vi "PicoLogHRDLGetSingleAsyncExample.vi"() -> ()   [LabVIEW 2010]
panel:
  out "maxAdc":i32
  out "Over Voltage":i16 format="%016b"
  out "handle":i16
  out "error out":errorcluster
  out "Unit Info":T1
  in  "range":i16=-1
  in  "channel":i16=-1
  in  "value":i32
  out "bStartedConversion":bool
  out "bConversionFinished":bool
  in  "stop":bool
  in  "error in (no error)":errorcluster
  out "Meter (mV)":dbl(knob)=-inf scale=-2500.0..2500.0
  in  "Input type":i16(ring)=1 items=["Differential", "Single-Ended"]
  in  "Conversion time":i16(ring)=4 items=["60ms", "100ms", "180ms", "340ms", "660ms"]
  in  "Voltage Range":i16(ring) items=["+/-2500mV", "+/-1200mV", "+/-625mV", "+/-312.5mV", "+/-156.25mV", "+/-78.125mV", "+/-39.0625mV"]
  in  "Channel":i16=1 min=1 max=16 step=1
  # "-1        if the unit fails to open\n0         if no unit is found\n>= 1   handle to the device opened"
  # "NOTES-\nNumber of channels-\nADC-20: 1 to 8\nADC-24: 1 to 16\n\nRange Voltage range Availability\n (0)    ±2500 mV        ADC-20 and ADC-24\n (1)    ±1250 mV        ADC-20 and ADC-24\n (2)    ±625 mV          ADC-24 only\n (3)    ±312.5 mV       ADC-24 only\n (4)    ±156.25 mV     ADC-24 only\n (5)    ±78.125 mV     ADC-24 only\n (6)    ±39.0625 mV   ADC-24 only"
  # "mV"
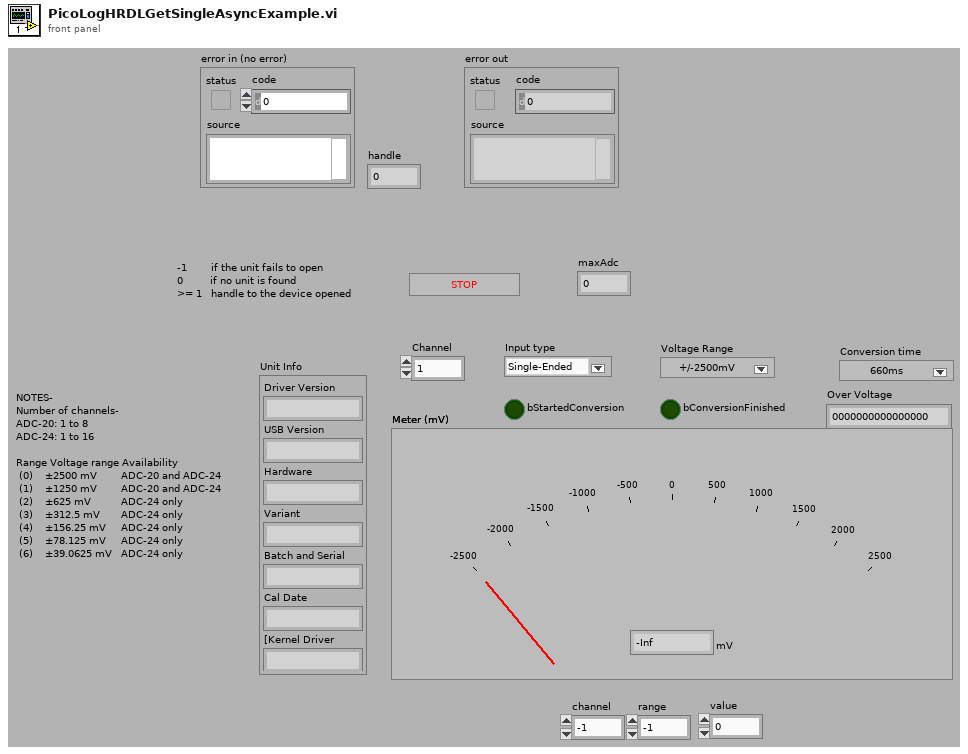
[diagram p1: front panel]
types:
  T1 = cluster{"Driver Version":string, "USB Version":string, "Hardware":string, "Variant":string, "Batch and Serial":string, "Cal Date":string, "[Kernel Driver":string, "[7]":string, "[8]":string, "[9]":string, "[10]":string, "[11]":string, "[12]":string, "[13]":string, "[14]":string}
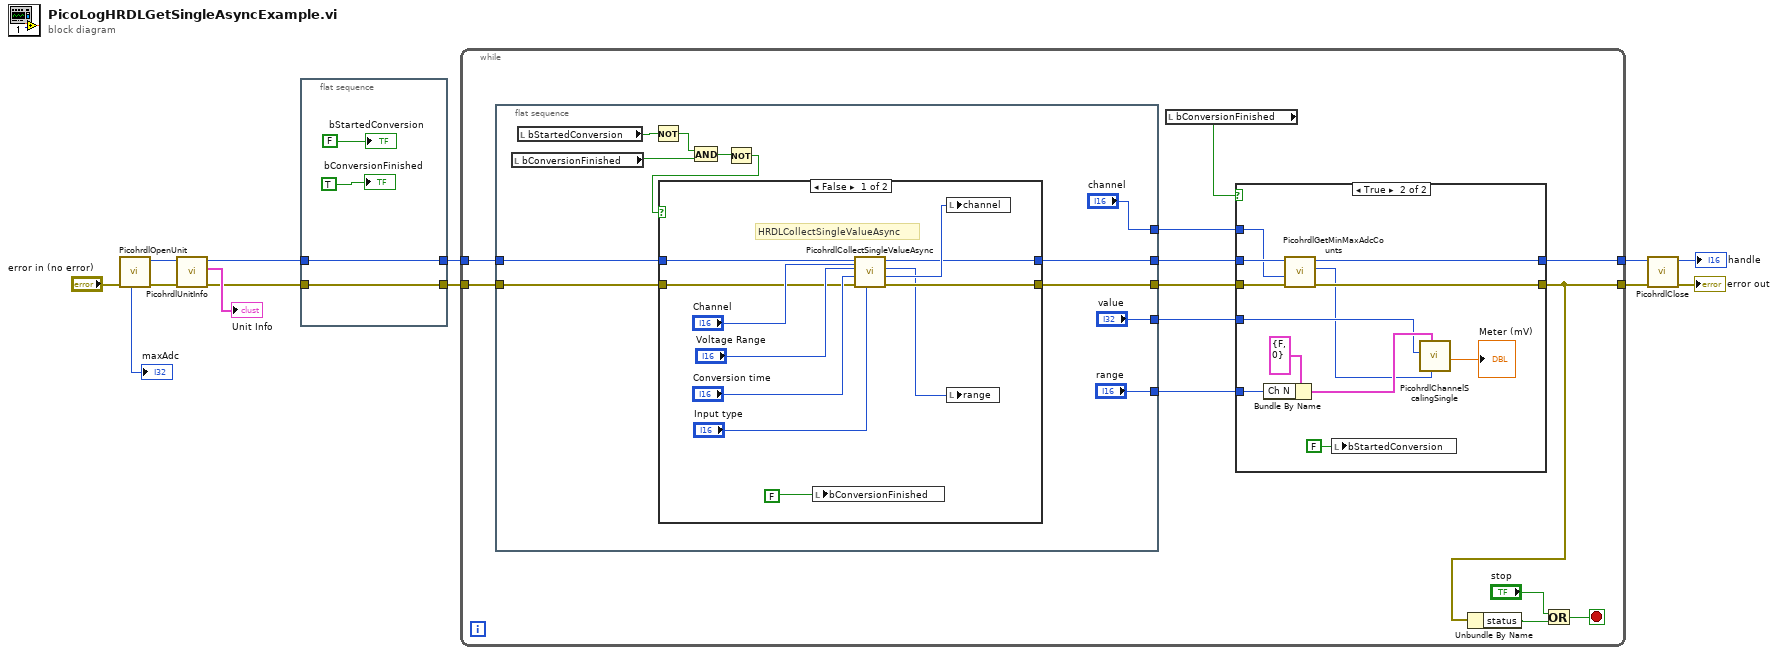
[diagram p0: block diagram]
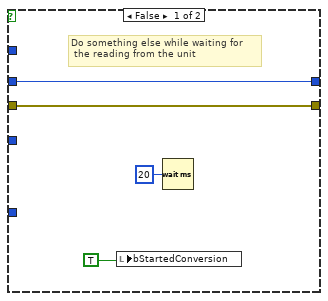
[diagram p2: hidden frame]
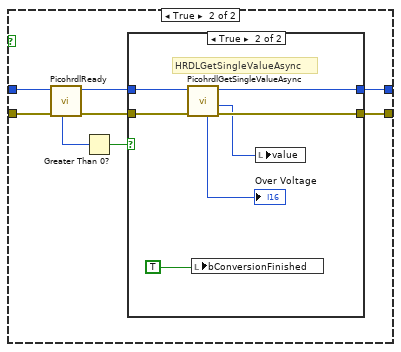
[diagram p3: hidden frame]
diagram:
  n1 = call "PicohrdlOpenUnit.vi"("error in (no error)"="error in (no error)") -> ("error out"=w11:errorcluster, "Handle out"=w10:i16, "maxAdc"=→"maxAdc":i32)  [unwired: 7 in, 1 out]
  n2 = call "PicohrdlUnitInfo.vi"("error in (no error)"=w11, "handle in"=w10) -> ("error out"=w4:errorcluster, "Unit Info"=→"Unit Info":T1, "handle out"=w2:i16)  [unwired: 7 in]
  n3 = flat-sequence {
    tunnel: [w15] -> w5
    tunnel: w4 -> [w15]
    tunnel: [w14] -> w3
    tunnel: w2 -> [w14]
    frame #0 {
      "bStartedConversion" <- FALSE ("bStartedConversion")
      "bConversionFinished" <- TRUE ("bConversionFinished")
    }
  }
  n4 = while {
    tunnel: w3 -> [w25]
    tunnel: [w23] -> w6
    tunnel: [w19] -> w7
    tunnel: w5 -> [w20]
    stop <- w28 stop-if-true
    n5 = flat-sequence {
      tunnel: ["range"] -> w27
      tunnel: ["value"] -> w26
      tunnel: w25 -> [w58]
      tunnel: [w57] -> w24
      tunnel: ["channel"] -> w22
      tunnel: [w56] -> w21
      tunnel: w20 -> [w55]
      frame #0 {
        n6 = local read "bConversionFinished"() -> (w51:bool)
        n7 = local read "bStartedConversion"() -> (w48:bool)
        n8 = Not(x=w48) -> (.not. x?=w47:bool)
        n9 = And(x=w47, y=w51) -> (x .and. y?=w50:bool)
        n10 = Not(x=w50) -> (.not. x?=w49:bool)
        n11 = case shown="False" w49 {
          tunnel: w58 -> [w60 w70]
          tunnel: [w61 w76] -> w57
          tunnel: [w64 w75] -> w56
          tunnel: w55 -> [w59 w74]
          frame False {
            # "HRDLCollectSingleValueAsync"
            n12 = local write "bConversionFinished"(FALSE ("bStartedConversion")) -> ()
            n13 = call "PicohrdlCollectSingleValueAsync.vi"("Input type"="Input type", "Channel in"="Channel", "error in (no error)"=w59, "Conversion time"="Conversion time", "Voltage Range"="Voltage Range", "handle in"=w60) -> ("error out"=w64:errorcluster, "channel"=w63:i16, "Voltage Range out"=w62:i16, "Handle out"=w61:i16)  [unwired: 2 in]
            n14 = local write "channel"(w63) -> ()
            n15 = local write "range"(w62) -> ()
          }
          frame True {
            n16 = call "PicohrdlReady.vi"("error in (no error)"=w74, "handle in"=w70) -> ("error out"=w73:errorcluster, "handle out"=w71:i16, "ready"=w72:i16)  [unwired: 7 in]
            n17 = Greater Than 0?(x=w72) -> (x > 0?=w77:bool)
            n18 = case shown="True" w77 {
              tunnel: w71 -> [w79 w84]
              tunnel: w73 -> [w78 w85]
              tunnel: [w79 w82] -> w76
              tunnel: [w78 w83] -> w75
              frame False {
                # "Unit still not ready"
              }
              frame True {
                # "HRDLGetSingleValueAsync"
                n19 = call "PicohrdlGetSingleValueAsync.vi"("error in (no error)"=w85, "handle in"=w84) -> ("error out"=w83:errorcluster, "value"=w80:i32, "Handle out"=w82:i16, "Over Voltage"=→"Over Voltage":i16)  [unwired: 6 in]
                n20 = local write "bConversionFinished"(TRUE ("bConversionFinished")) -> ()
                n21 = local write "value"(w80) -> ()
              }
            }
          }
        }
      }
    }
    n22 = local read "bConversionFinished"() -> (w30:bool)
    n23 = case shown="True" w30 {
      tunnel: w27 -> [_ w44]
      tunnel: w26 -> [_ w42]
      tunnel: w24 -> [w34 w40]
      tunnel: [w34 w36] -> w23
      tunnel: w22 -> [_ w38]
      tunnel: [w33 w37] -> w19
      tunnel: w21 -> [w33 w39]
      frame False {
        # "Do something else while waiting for\n the reading from the unit"
        n24 = local write "bStartedConversion"(TRUE ("bStartedConversion")) -> ()
        n25 = Wait (ms)(milliseconds to wait=u32 20) -> ()  [unwired: 1 out]
      }
      frame True {
        n26 = Bundle By Name(cluster=cluster{bool, "Ch N":i16} {FALSE, "Ch N"=0} ("input cluster"), "Ch N"=w44) -> (w43:cluster{bool, "Ch N":i16})
        n27 = call "PicohrdlGetMinMaxAdcCounts.vi"("error in (no error)"=w39, "channel"=w38, "handle in"=w40) -> ("error out"=w37:errorcluster, "maxAdc"=w35:i32, "handle out"=w36:i16)  [unwired: 5 in, 1 out]
        n28 = local write "bStartedConversion"(FALSE ("bStartedConversion")) -> ()
        n29 = call "PicohrdlChannelScalingSingle.vi"("Max_adc"=w35, "Channel N"=w43, "DataIn"=w42) -> ("DataOut"=→"Meter (mV)":dbl)  [unwired: 8 in]
      }
    }
    n30 = Unbundle By Name(w19) -> ("status"=w18:bool)
    n31 = Or(x="stop", y=w18) -> (x .or. y?=w28:bool)
  }
  n32 = call "PicohrdlClose.vi"("error in (no error)"=w7, "Handle in"=w6) -> ("error out"=→"error out":errorcluster, "handle"=→"handle":i16)  [unwired: 8 in]
